vi "DoTeleop-C.vi"(11 "Params":string[][](array[string])) -> ()   [LabVIEW 2018]
uses:
  <vilib>/Rock Robotics/WPI/DriverStation/WPI_DriverStationDerivedRobotMode.ctl
  Framework/Robot Global Data.vi
  <vilib>/Rock Robotics/WPI/Utilities/WPI_GetSetVariantRefNum.vi
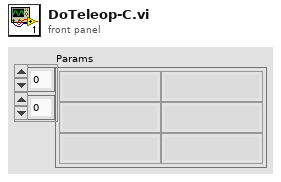
[diagram p1: front panel]
types:
  T1 = typedef "WPI_DriverStationDerivedRobotMode.ctl" = enum16{"Init", "Execute", "Stop"}
  T2 = typedef "WPI_JoystickDevRef.ctl" = cluster{"Device":T3}
  T3 = typedef "WPI_JoystickDeviceEnum.ctl" = enum16{"USB 0", "USB 1", "USB 2", "USB 3", "USB 4", "USB 5"}
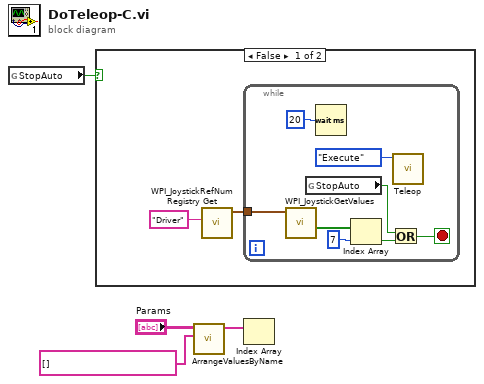
[diagram p0: block diagram]
diagram:
  n1 = global read "Robot Global Data.vi" "StopAuto"() -> (w4:bool)
  n2 = case shown="False" w4 {
    frame False {
      n3 = call <vilib>:"WPI_JoystickRefNum Registry Get.vi"("refnum name"="Driver") -> ("JoystickDevRef"=w5:T2)  [unwired: 9 in, 1 out]
      n4 = while {
        tunnel: w5 -> [w14]
        stop <- w8 stop-if-true
        n5 = call <vilib>:"WPI_JoystickGetValues.vi"("JoystickDevRef"=w14) -> ("Buttons"=w12:bool[])  [unwired: 6 in, 4 out]
        n6 = global read "Robot Global Data.vi" "StopAuto"() -> (w9:bool)
        n7 = Wait (ms)(milliseconds to wait=u32 20) -> ()  [unwired: 1 out]
        n8 = Index Array(array=w12, index=7) -> (element=w10:bool)
        n9 = Or(x=w9, y=w10) -> (x .or. y?=w8:bool)
        n10 = call "Teleop.vi"("Call Context"=WPI_DriverStationDerivedRobotMode."Execute") -> ()  [unwired: 11 in]
      }
    }
    frame True {
    }
  }
  n11 = call "ArrangeValuesByName.vi"("Names"=string[] [], "Names/Values in"="Params") -> ("Values Out"=w1:string[])  [unwired: 9 in]
  n12 = Index Array(array=w1) -> ()  [unwired: 1 in, 1 out]
